vi "Msg Handler.vi"(10 "Msg":refnum<class "Msg.lvclass">, 11 "Base Actor in":refnum<class "Base Actor.lvclass">) -> (0 "Error out":errorcluster, 3 "Base Actor out":refnum<class "Base Actor.lvclass">)   [LabVIEW 2025, in "jettl.lvlib" / "Actor.lvlib" / "Base Actor.lvclass"]
uses:
  Base Actor.lvclass
  C:/git/jettl/src/jettl/jettl/Actor/Actor/Actor.lvclass
  Msg/Msg.lvclass
  Base Actor.lvclass/Base Actor.ctl
  Actor.lvlib
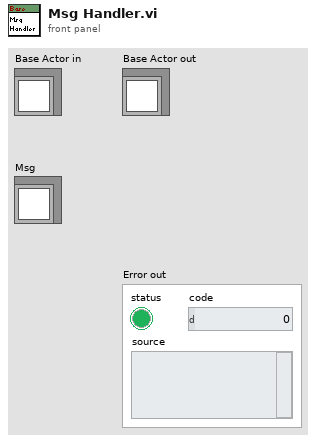
[diagram p1: front panel]
types:
  T1 = typedef "jettl.lvlib/Actor.lvlib/Msg Set.ctl" = set{refnum<class "Msg.lvclass">}
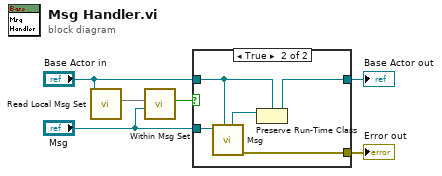
[diagram p0: block diagram]
diagram:
  n1 = call-dynamic "Read Local Msg Set.vi"("Base Actor in"="Base Actor in") -> ("Local Msg Set"=w1:T1)  [unwired: 10 in]
  n2 = call "Within Msg Set.vi"("Msg"="Msg", "Msg Set"=w1) -> ("Within Msg Set"=w6:bool)  [unwired: 9 in]
  n3 = case shown="True" w6 {
    tunnel: "Base Actor in" -> [w7 w10]
    tunnel: [w7 w9] -> w5
    tunnel: "Msg" -> [_ w12]
    tunnel: [_ w8] -> w3
    frame False {
      # "This is the inner most layer, do nothing."
    }
    frame True {
      n4 = call-dynamic "Msg.vi"("Actor in"=w10, "Msg in"=w12) -> ("Error out"=w8:errorcluster, "Actor out"=w11:refnum<class "Actor.lvclass">)  [unwired: 8 in]
      n5 = Preserve Run-Time Class(object in=w11, 2:w10) -> (object out=w9:refnum<class "Base Actor.lvclass">)  [unwired: 1 in, 1 out]
    }
  }
  "Base Actor out" <- w5
  "Error out" <- w3
